vi "Image-correction.vi"(8 "error in":errorcluster, 9 "Correct. params. ref. in":refnum<data-value>, 10 "Buffer element in":T1 {"Temperature characteristics"."Stand. dev. temperature" format="%#.1f"; "Temperature characteristics"."Min. temperature" format="%#.0f"; "Temperature characteristics"."Max. temperature" format="%#.0f"; "Temperature characteristics"."Average temperature" format="%#.0f"}, 11 "Buffers in":refnum<class "CV-Buffers.lvclass">) -> (0 "error IO":errorcluster, 1 "Correct. params. ref.":refnum<data-value>, 2 "Buffer element":T1 {"Temperature characteristics"."Stand. dev. temperature" format="%#.1f"; "Temperature characteristics"."Min. temperature" format="%#.0f"; "Temperature characteristics"."Max. temperature" format="%#.0f"; "Temperature characteristics"."Average temperature" format="%#.0f"}, 3 "Buffers":refnum<class "CV-Buffers.lvclass">)   [LabVIEW 2013, in "CameraVision.lvlib" / "CV-Main.lvclass"]
uses:
  CV-Main.lvclass
  Correction/CV-Correction.lvclass
  Buffers/Storage-buffer.ctl
  <vilib>/vision/Image Controls.llb/IMAQ Image.ctl
  Temperature/Temperature-characteristics.ctl
  Analysis/Characteristics-cluster.ctl
  Buffers/CV-Buffers.lvclass
  Buffers/CV-Buffers.lvclass/CV-Buffers.ctl
  Correction/CV-Correction.lvclass/CV-Correction.ctl
  Correction/Read Background correction type.vi
  Buffers/Read Black image refs.vi
  <vilib>/vision/NI_Vision_Development_Module.lvlib
  Temperature/CV-Temperature.lvclass
  Analysis/CV-Analysis.lvclass
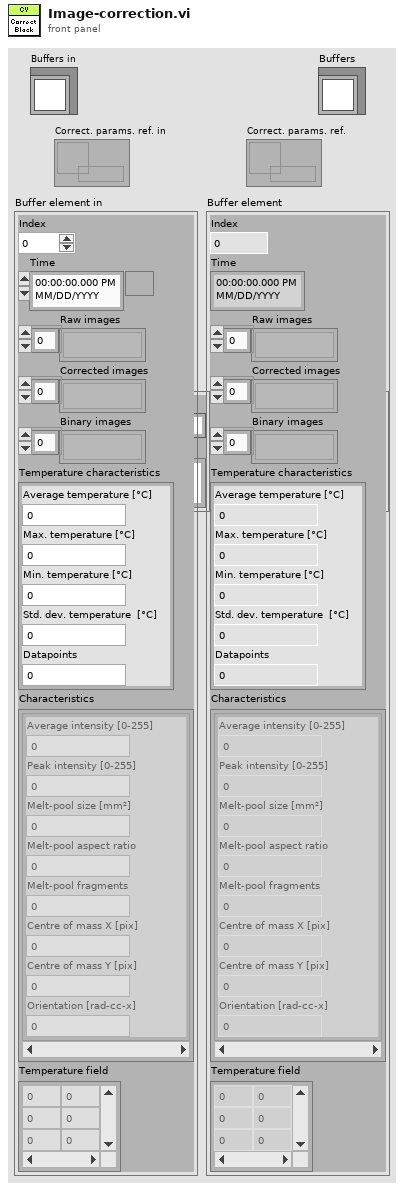
[diagram p1: front panel]
types:
  T1 = typedef "CameraVision.lvlib/CV-Buffers.lvclass/Storage-buffer.ctl" = cluster{"Index":i32, "Time":timestamp, "Raw images":T2[], "Corrected images":T2[], "Binary images":T2[], "Temperature characteristics":T3, "Characteristics":T4[], "Temperature field":dbl[][]}
  T2 = typedef "IMAQ Image.ctl" = refnum<image>
  T3 = typedef "CameraVision.lvlib/CV-Temperature.lvclass/Temperature-characteristics.ctl" = cluster{"Average temperature ":dbl, "Max. temperature":dbl, "Min. temperature":dbl, "Stand. dev. temperature":dbl, "Datapoints":dbl}
  T4 = typedef "CameraVision.lvlib/CV-Analysis.lvclass/Characteristics-cluster.ctl" = cluster{"Average intensity":dbl, "Peak intensity":dbl, "Melt-pool size":dbl, "Melt-pool aspect ratio":dbl, "Melt-pool fragments":dbl, "Centre of mass X":dbl, "Centre of mass Y":dbl, "Orientation":dbl}
  T5 = typedef "CameraVision.lvlib/Correction.lvclass/Background-correction.ctl" = enum16{"Hardware", "Software"}
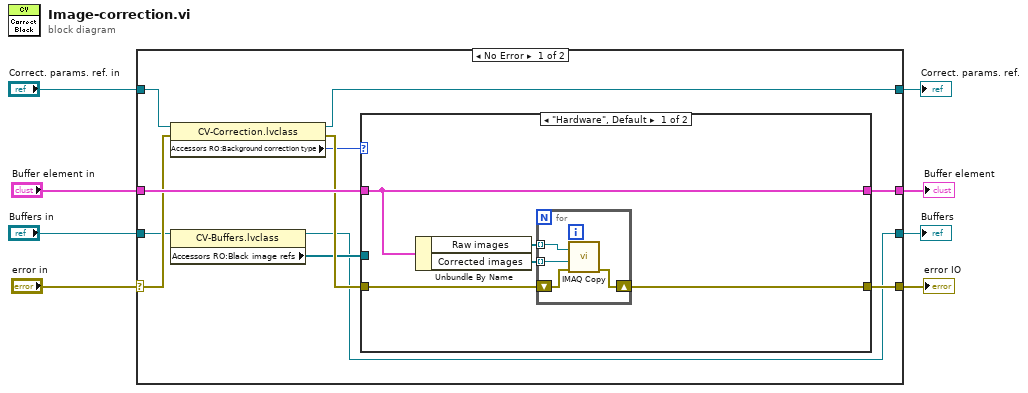
[diagram p0: block diagram]
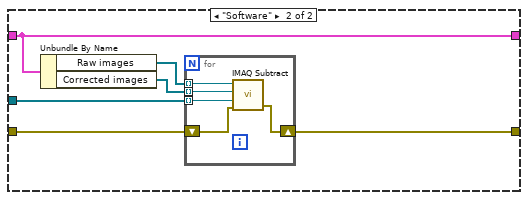
[diagram p2: hidden frame]
diagram:
  n1 = case shown="No Error" "error in" {
    selector: "error in" -> [w17 w43]
    tunnel: [w18 w43] -> w7
    tunnel: "Buffer element in" -> [w19 w41]
    tunnel: "Correct. params. ref. in" -> [w14 w42]
    tunnel: [w15 w42] -> w4
    tunnel: [w12 w41] -> w3
    tunnel: "Buffers in" -> [w11 w40]
    tunnel: [w9 w40] -> w1
    frame No Error {
      n2 = property class="CV-Correction.lvclass"(reference=w14, error in=w17) -> (reference out=w15:refnum<data-value>, error out=w16:errorcluster, "Accessors RO:Background correction type"=w13:T5)
      n3 = property class="CV-Buffers.lvclass"(reference=w11) -> (reference out=w9:refnum<class "CV-Buffers.lvclass">, "Accessors RO:Black image refs"=w10:T2[])  [unwired: 1 in, 1 out]
      n4 = case shown="\"Hardware\", Default" w13 {
        tunnel: w19 -> [w20 w31]
        tunnel: w16 -> [w22 w33]
        tunnel: [w21 w32] -> w18
        tunnel: [w20 w31] -> w12
        tunnel: w10 -> [_ w30]
        frame "Hardware", Default {
          n5 = Unbundle By Name(w20) -> ("Raw images"=w24:T2[], "Corrected images"=w23:T2[])
          n6 = for {
            tunnel: w24 -> [w28] mode=indexing
            tunnel: w23 -> [w27] mode=indexing
            shift-right: [w25] -> w21
            shift-left: w22 -> [w26]
            n7 = call "IMAQ Copy"("error in (no error)"=w26, "Image Dst"=w27, "Image Src"=w28) -> ("error out"=w25:errorcluster)  [unwired: 3 in, 1 out]
          }
        }
        frame "Software" {
          n8 = Unbundle By Name(w31) -> ("Raw images"=w34:T2[], "Corrected images"=w29:T2[])
          n9 = for {
            tunnel: w34 -> [w39] mode=indexing
            tunnel: w30 -> [w38] mode=indexing
            tunnel: w29 -> [w37] mode=indexing
            shift-right: [w36] -> w32
            shift-left: w33 -> [w35]
            n10 = call "IMAQ Subtract"("Image Src A"=w39, "Image Dst"=w37, "Image Src B"=w38, "error in (no error)"=w35) -> ("error out"=w36:errorcluster)  [unwired: 3 in, 1 out]
          }
        }
      }
    }
    frame Error {
    }
  }
  "error IO" <- w7
  "Buffer element" <- w3
  "Correct. params. ref." <- w4
  "Buffers" <- w1
